vi "OCU_Simple_Main.vi"() -> ()   [LabVIEW 2013]
doc: "To be executed on the Opperator Control Unit (laptop), which communicates to a variety of platforms for the sailbot boat to send missions to complete, override commands, and to monitor the status of the boat and parts of the code run on it. It should be run in parallel with \"Main.vi\" in the cRIO code foler. \n\nCreaded by Victoria Coleman and Elizabeth Mahon (03/14)"
uses:
  cRIO_Code/Data/TypeDefs/UTM Location.ctl
  cRIO_Code/Data/TypeDefs/Constants for OCU Tuning.ctl
  cRIO_Code/Data/TypeDefs/MotorSetup.ctl
  cRIO_Code/Data/TypeDefs/DynamixelSetupInfo.ctl
  cRIO_Code/Data/TypeDefs/Sail Set Suggestions.ctl
  cRIO_Code/Data/TypeDefs/Rudder Set Suggestions.ctl
  cRIO_Code/Logic/Classes/Missions/GenericMission/GenericMission.lvclass
  cRIO_Code/Data/TypeDefs/MainsailPositionIndicator.ctl
  cRIO_Code/Data/TypeDefs/JibPositionIndicator.ctl
  cRIO_Code/Data/TypeDefs/Apparent Wind Point of Sail.ctl
  cRIO_Code/Data/TypeDefs/BoatType.ctl
  cRIO_Code/Logic/Classes/Waypoint/Waypoint.lvclass
  cRIO_Code/Data/TypeDefs/MissionDescription.ctl
  cRIO_Code/Data/TypeDefs/MissionTypeControl.ctl
  cRIO_Code/Data/TypeDefs/Sim_Wind_Speed.ctl
  cRIO_Code/Data/TypeDefs/Sim_Wind_Heading.ctl
  cRIO_Code/Data/TypeDefs/OverrideInformation.ctl
  cRIO_Code/Data/TypeDefs/OverrideMode.ctl
  TypeDef/map_list.ctl
  TypeDef/obstacle_arrays.ctl
  cRIO_Code/Logic/Classes/Obstacle/Obstacle.lvclass
  cRIO_Code/Data/TypeDefs/ObstacleDescription.ctl
  CommandMessages.ctl
  cRIO_Code/Logic/Classes/Missions/GoTo/GoTo.lvclass
  RIO-OCU_Comm/NetworkStreams/Writer/NetworkStreamWriter.lvclass
  RIO-OCU_Comm/NetworkStreams/Reader/NetworkStreamReader.lvclass
panel:
  in  "Main Tab Structure":enum32{"User Interface", "Settings"}(tab)
  in  "Setting Missions with Map Internal Tab":enum32{"Edit Mission", "Monitor Boat"}(tab)
  in  "element":T1 {"North" format="%#_10f"; "East" format="%#_8f"}
  in  "ClearMissionPOI":bool
  in  "CreateMission":bool
  out "Readable Missions":T2[](array[typedef]) {"Points of Interest"."North" format="%#_10f"; "Points of Interest"."East" format="%#_8f"}
  out "Robot Location":T1 {"North" format="%#_10f"; "East" format="%#_8f"}
  out "Rudder Setpoint":T4 min=-0.95 max=0.95 scale=1.0..-1.0
  out "BoatSpeed":dbl(slide) scale=0.0..100.0
  out "Abs Wind Direction":dbl(knob)
  out "Main":T5
  out "Jib":T6
  out "BoatDirection":dbl(knob)
  out "RelWindDirection":T7 scale=0.0..360.0 scale format="%4d"
  out "Set Mission with Map":T8(plugin-control)
  in  "Sim_Wind_Heading":T9
  in  "Sim_Wind_Speed":T10
  out "Reset missions?":bool=TRUE
  out "Missions from Main":refnum<class "GenericMission.lvclass">[](array[class])
  out "Current Missions":refnum<class "GenericMission.lvclass">[](array[class])
  out "Finished Missions":refnum<class "GenericMission.lvclass">[](array[class])
  out "Map display loop counter":i32
  out "User input loop counter":i32
  out "Desired Heading":dbl
  out "Abs Wind Direction":dbl(knob)
  out "Rel Wind Direction":dbl(knob)
  out "Sail Positions":T11 {"MainSailSuggestion" min=0.0 max=1.0; "JibSailSuggestion" min=0.0 max=1.0}
  out "Rudder Setpoint":T4 min=-0.95 max=0.95 scale=1.0..-1.0
  out "BoatDirection":dbl
  out "Final error out":errorcluster
  out "Intermediate\nWaypoints":refnum<class "Waypoint.lvclass">[](array[class])
  in  "Boat Type":T12
  in  "OCU Tuning Constants":T13={"Motor Setting Constant"={"Main Dynamixel Set Data"={"Lower Winch Bound (deg)"=0.0, "Upper Winch Bound (deg)"=1000.0}, "Rudder Dynamixel Set Data"={"Lower Winch Bound (deg)"=30.0, "Upper Winch Bound (deg)"=90.0}, "Jib Dynamixel Set Data"={"Lower Winch Bound (deg)"=0.0, "Upper Winch Bound (deg)"=700.0}}, "Irons Range (deg)"=100.0}
  out "Reader\nConnected?":bool
  out "Writter\nConnected?":bool
  in  "Clear Trace":bool
  in  "Trace Path":bool=TRUE
  out "Sending IDs?":bool
  out "Mission Points of Interest":T1[](array[typedef]) {"North" format="%#_10f"; "East" format="%#_8f"}
  in  "ID# To Delete (miss)":u16
  in  "DeleteMission":bool
  in  "stop":bool
  # "These guys need to be kept even though they aren't human readable, they're used for probing and data passage"
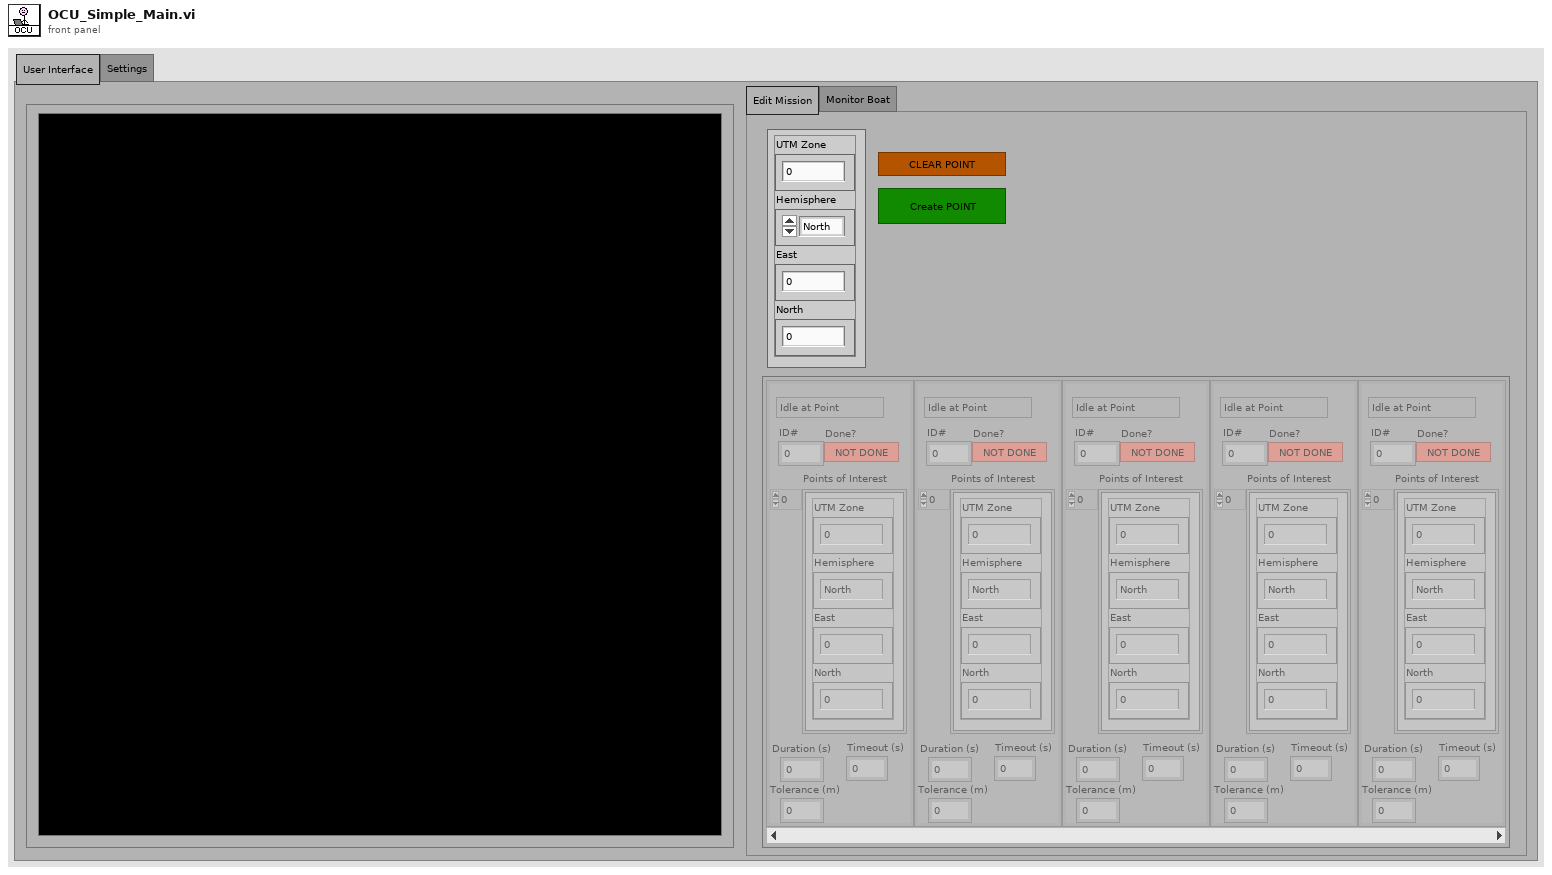
[diagram p1: front panel]
types:
  T1 = typedef "UTM Location.ctl" = cluster{"UTM Zone":dbl, "Hemisphere":enum16{"North", "South"}, "East":dbl, "North":dbl}
  T2 = typedef "MissionDescription.ctl" = cluster{"Duration (s)":dbl, "Timeout (s)":dbl, "Tolerance (m)":dbl, "Mission Type":T3, "Points of Interest":T1[], "ID#":i32, "Done?":bool}
  T3 = typedef "MissionTypeControl.ctl" = enum16{"Idle at Point", "Drive to Waypoint", "Round Buoy to Port", "Round Buoy to Starboard", "Pass Between Buoys", "Station Keeping"}
  T4 = typedef "Rudder Set Suggestions.ctl" = dbl
  T5 = typedef "MainsailPositionIndicator.ctl" = dbl
  T6 = typedef "JibPositionIndicator.ctl" = dbl
  T7 = typedef "Apparent Wind Point of Sail.ctl" = dbl
  T8 = typedef "IMAQ Image.ctl" = refnum<image>
  T9 = typedef "Sim_Wind_Heading.ctl" = dbl
  T10 = typedef "Sim_Wind_Speed.ctl" = dbl
  T11 = typedef "Sail Set Suggestions.ctl" = cluster{"MainSailSuggestion":dbl, "JibSailSuggestion":dbl}
  T12 = typedef "BoatType.ctl" = enum16{"Blackbody Radiation", "ReadLog", "Little boats", "Simulation", "Damn Yankee"}
  T13 = typedef "Constants for OCU Tuning.ctl" = cluster{"Motor Setting Constant":T14, "Irons Range (deg)":dbl}
  T14 = typedef "MotorSetup.ctl" = cluster{"Main Dynamixel Set Data":T15, "Rudder Dynamixel Set Data":T15, "Jib Dynamixel Set Data":T15}
  T15 = typedef "DynamixelSetupInfo.ctl" = cluster{"Lower Winch Bound (deg)":dbl, "Upper Winch Bound (deg)":dbl}
  T16 = typedef "map_list.ctl" = enum16{"Grid", "Olin"}
  T17 = typedef "OverrideInformation.ctl" = cluster{"OverrideMode":T18, "SailSetting":T11, "Rudder Setpoint":T4, "Sim_Wind_Speed":dbl, "Sim_Wind_Heading":dbl}
  T18 = typedef "OverrideMode.ctl" = enum16{"None", "Rudder", "Sails", "Both"}
  T19 = typedef "mission_arrays.ctl" = cluster{"# of Missions":i32, "Readable Missions":T2[], "Mission array":refnum<class "GenericMission.lvclass">[]}
  T20 = typedef "map_metadata.ctl" = cluster{"Meters/pixel":dbl, "Top Left Pixel UTM":T1, "Bottom Right Pixel UTM":T1}
  T21 = typedef "obstacle_arrays.ctl" = cluster{"# of Obstacles":i32, "Obstacle array":refnum<class "Obstacle.lvclass">[], "Readable Obstacles":T22[]}
  T22 = typedef "ObstacleDescription.ctl" = cluster{"ID#":i32, "Obstacle Array":T1[]}
  T23 = typedef "CommandMessages.ctl" = enum16{"Pass", "OverrideMode", "Add mission", "Delete mission", "Add obstacle", "Delete obstacle", "Change constants", "Check mission ID", "Check obstacle ID"}
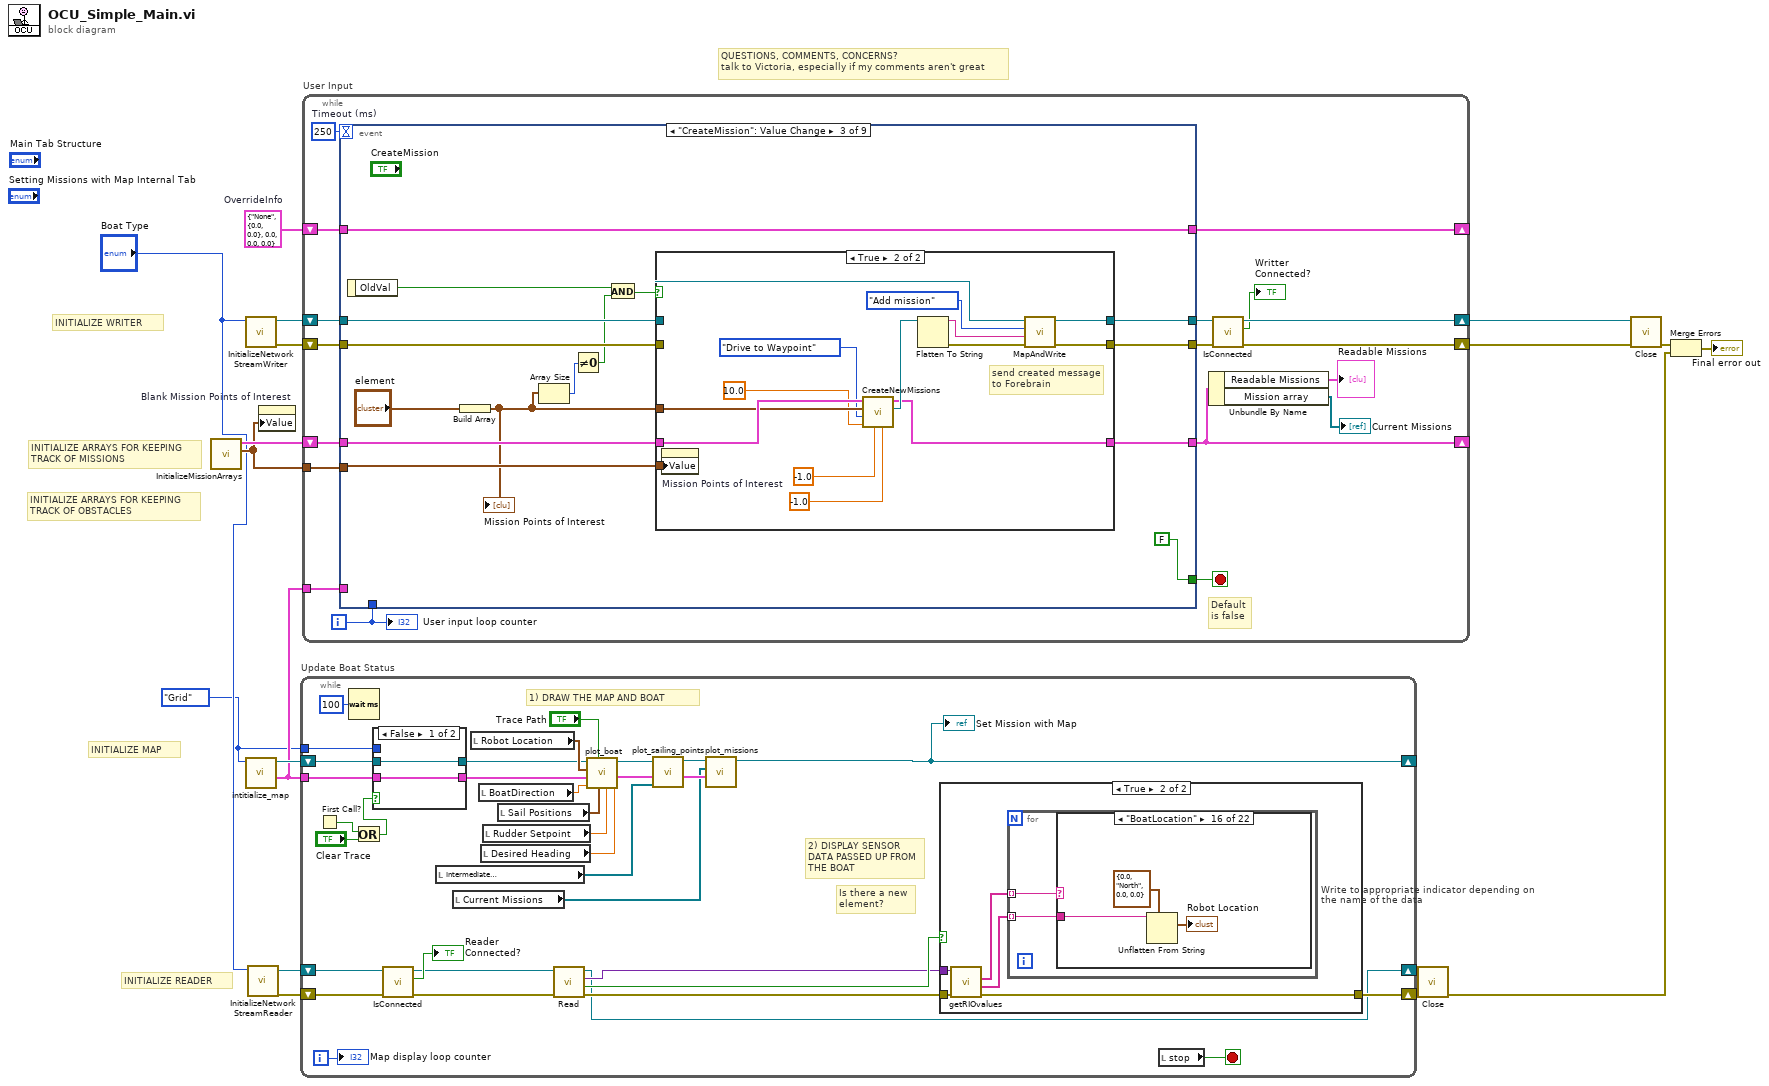
[diagram p0: block diagram]
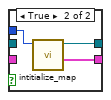
[diagram p2: hidden frame]
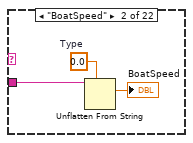
[diagram p5: hidden frame]
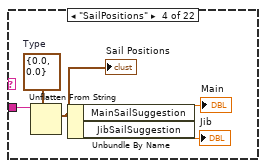
[diagram p7: hidden frame]
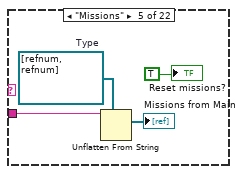
[diagram p8: hidden frame]
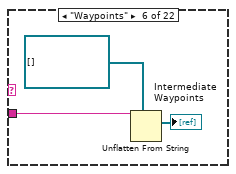
[diagram p9: hidden frame]
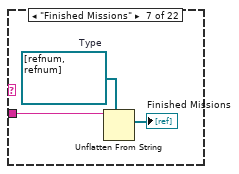
[diagram p10: hidden frame]
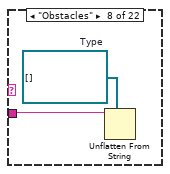
[diagram p11: hidden frame]
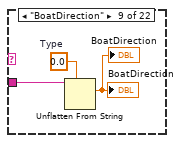
[diagram p12: hidden frame]
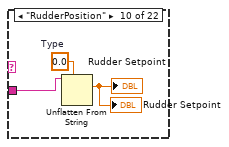
[diagram p13: hidden frame]
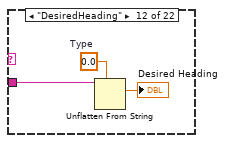
[diagram p15: hidden frame]
diagram:
  w1 = map_list."Grid" ("Map")
  w5 = T17 {"OverrideMode"=enum."None", "SailSetting"={"MainSailSuggestion"=0.0, "JibSailSuggestion"=0.0}, "Rudder Setpoint"=0.0, "Sim_Wind_Speed"=0.0, "Sim_Wind_Heading"=0.0}  # OverrideInfo
  # "INITIALIZE ARRAYS FOR KEEPING TRACK OF OBSTACLES"
  # "INITIALIZE WRITER"
  # "INITIALIZE ARRAYS FOR KEEPING TRACK OF MISSIONS"
  # "INITIALIZE MAP"
  # "INITIALIZE READER"
  # "QUESTIONS, COMMENTS, CONCERNS? \ntalk to Victoria, especially if my comments aren't great"
  n1 = call "InitializeMissionArrays.vi"() -> ("Mission Points of Interest"=w3:T1[], "Initialized Mission Arrays"=w18:T19)  [unwired: 10 in]
  n2 = call "InitializeNetworkStreamWriter.vi"("Boat Type"="Boat Type") -> ("error out"=w15:errorcluster, "NetworkStreamWriter out"=w14:refnum<class "NetworkStreamWriter.lvclass">)  [unwired: 9 in]
  n3 = call "intitialize_map.vi"("Map"=w1) -> ("MapDistanceInfo"=w4:T20, "Map Image Out"=w11:T8)  [unwired: 9 in]
  n4 = call "InitializeNetworkStreamReader.vi"("Boat Type"="Boat Type") -> ("error out"=w9:errorcluster, "NetworkStreamReader out"=w10:refnum<class "NetworkStreamReader.lvclass">)  [unwired: 9 in]
  n5 = property on="Blank Mission Points of Interest" class="Arr (strict)"("Value"=w3) -> ()  [unwired: 2 in, 2 out]
  n6 = while "Update Boat Status" {
    shift-right: [w41] -> w13
    shift-left: w10 -> [w51]
    shift-right: [w47] -> w12
    shift-left: w9 -> [w50]
    tunnel: w4 -> [w36]
    tunnel: w1 -> [w38]
    shift-right: [w23] -> _
    shift-left: w11 -> [w39]
    i -> [w37]
    stop <- w52 stop-if-true
    # "Is there a new element?"
    # "2) DISPLAY SENSOR DATA PASSED UP FROM THE BOAT"
    # "1) DRAW THE MAP AND BOAT"
    n7 = First Call?() -> (First Call?: T/F=w26:bool)
    n8 = Wait (ms)(milliseconds to wait=u32 100) -> ()  [unwired: 1 out]
    n9 = Or(x=w26, y="Clear Trace") -> (x .or. y?=w25:bool)
    n10 = case shown="False" w25 {
      tunnel: w39 -> [w54 _]
      tunnel: [w54 w55] -> w28
      tunnel: w36 -> [w53 _]
      tunnel: [w53 w56] -> w29
      tunnel: w38 -> [_ w57]
      frame False {
      }
      frame True {
        n11 = call "intitialize_map.vi"("Map"=w57) -> ("MapDistanceInfo"=w56:T20, "Map Image Out"=w55:T8)  [unwired: 9 in]
      }
    }
    n12 = call "IsConnected.vi"("error in (no error)"=w50, "NetworkStreamReader in"=w51) -> ("error out"=w45:errorcluster, "Connected?"=→"Reader\nConnected?":bool, "NetworkStreamReader out"=w46:refnum<class "NetworkStreamReader.lvclass">)  [unwired: 7 in]
    n13 = local read "Intermediate\nWaypoints"() -> (w22:refnum<class "Waypoint.lvclass">[])
    n14 = local read "Current Missions"() -> (w19:refnum<class "GenericMission.lvclass">[])
    n15 = local read "Robot Location"() -> (w32:T1)
    n16 = local read "BoatDirection"() -> (w34:dbl)
    n17 = local read "Desired Heading"() -> (w24:dbl)
    n18 = local read "Rudder Setpoint"() -> (w33:T4)
    n19 = local read "Sail Positions"() -> (w35:T11)
    n20 = call "Read.vi"("error in (no error)"=w45, "NetworkStreamReader in"=w46) -> ("error out"=w44:errorcluster, "New element?"=w43:bool, "element"=w42:variant, "NetworkStreamReader out"=w41:refnum<class "NetworkStreamReader.lvclass">)  [unwired: 5 in, 1 out]
    n21 = call "plot_boat.vi"("Desired Heading"=w24, "Rudder Setpoint"=w33, "Sail Setpoints"=w35, "Trace Path"="Trace Path", "Heading"=w34, "MapDistanceInfo"=w29, "UTM Location"=w32, "Map in"=w28) -> ("MapDistanceInfo OUT"=w30:T20, "Map Out"=w31:T8)  [unwired: 1 in, 1 out]
    n22 = call "plot_sailing_points.vi"("Intermediate\nWaypoints"=w22, "MapDistanceInfo"=w30, "Map in"=w31) -> ("MapDistanceInfo OUT"=w21:T20, "Map Out"=w20:T8)  [unwired: 6 in, 1 out]
    n23 = call "plot_missions.vi"("MapDistanceInfo"=w21, "Missions"=w19, "Map in"=w20) -> ("Map Out"=w23:T8)  [unwired: 6 in, 2 out]
    "Set Mission with Map" <- w23
    n24 = case shown="True" w43 {
      tunnel: [w58 w61] -> w47
      tunnel: w44 -> [w58 w60]
      tunnel: w42 -> [_ w59]
      frame False {
      }
      frame True {
        n25 = call "getRIOvalues.vi"("error in"=w60, "element"=w59) -> ("error out"=w61:errorcluster, "data"=w62:string[], "names"=w63:string[])  [unwired: 7 in]
        n26 = for "Write to appropriate indicator depending on the name of the data" {
          tunnel: w63 -> [w65] mode=indexing
          tunnel: w62 -> [w64] mode=indexing
          n27 = case shown="\"BoatLocation\"" w65 {
            tunnel: w64 -> [_ w66 _ w73 w76 w80 w83 w84 w88 w91 _ w92 _ _ _ w97 _ _ _ w99 w103 _]
            frame Default {
              # "unknown name"
            }
            frame "BoatSpeed" {
              w68 = 0.0  # Type
              n28 = Unflatten From String(type=w68, binary string=w66) -> (value=→"BoatSpeed":dbl)  [unwired: 3 in, 2 out]
            }
            frame "WindSpeed" {
            }
            frame "SailPositions" {
              w72 = T11 {"MainSailSuggestion"=0.0, "JibSailSuggestion"=0.0}  # Type
              n29 = Unflatten From String(type=w72, binary string=w73) -> (value=w71:T11)  [unwired: 3 in, 2 out]
              "Sail Positions" <- w71
              n30 = Unbundle By Name(w71) -> ("MainSailSuggestion"=→"Main":dbl, "JibSailSuggestion"=→"Jib":dbl)
            }
            frame "Missions" {
              w77 = refnum<class "GenericMission.lvclass">[] [refnum, refnum]  # Type
              n31 = Unflatten From String(type=w77, binary string=w76) -> (value=→"Missions from Main":refnum<class "GenericMission.lvclass">[])  [unwired: 3 in, 2 out]
              "Reset missions?" <- TRUE
            }
            frame "Waypoints" {
              n32 = Unflatten From String(type=refnum<class "Waypoint.lvclass">[] [] ("elements"), binary string=w80) -> (value=→"Intermediate\nWaypoints":refnum<class "Waypoint.lvclass">[])  [unwired: 3 in, 2 out]
            }
            frame "Finished Missions" {
              w82 = refnum<class "GenericMission.lvclass">[] [refnum, refnum]  # Type
              n33 = Unflatten From String(type=w82, binary string=w83) -> (value=→"Finished Missions":refnum<class "GenericMission.lvclass">[])  [unwired: 3 in, 2 out]
            }
            frame "Obstacles" {
              w85 = refnum<class "Obstacle.lvclass">[] []  # Type
              n34 = Unflatten From String(type=w85, binary string=w84) -> ()  [unwired: 3 in, 3 out]
            }
            frame "BoatDirection" {
              w87 = 0.0  # Type
              n35 = Unflatten From String(type=w87, binary string=w88) -> (value=→"BoatDirection" →"BoatDirection":dbl)  [unwired: 3 in, 2 out]
            }
            frame "RudderPosition" {
              w90 = T4 0.0  # Type
              n36 = Unflatten From String(type=w90, binary string=w91) -> (value=→"Rudder Setpoint" →"Rudder Setpoint":T4)  [unwired: 3 in, 2 out]
            }
            frame "SimWindSpeed(m/s)" {
            }
            frame "DesiredHeading" {
              w94 = 0.0  # Type
              n37 = Unflatten From String(type=w94, binary string=w92) -> (value=→"Desired Heading":dbl)  [unwired: 3 in, 2 out]
            }
            frame "RudderForce" {
            }
            frame "BatteryVoltage" {
            }
            frame "StayForces" {
            }
            frame "BoatLocation" {
              n38 = Unflatten From String(type=T1 {"UTM Zone"=0.0, "Hemisphere"=enum."North", "East"=0.0, "North"=0.0} ("UTM Location"), binary string=w97) -> (value=→"Robot Location":T1)  [unwired: 3 in, 2 out]
            }
            frame "Pitch" {
            }
            frame "Roll" {
            }
            frame "RateOfTurn" {
            }
            frame "RelWindDirection" {
              w100 = 0.0  # Type
              n39 = Unflatten From String(type=w100, binary string=w99) -> (value=→"Rel Wind Direction" →"RelWindDirection":dbl)  [unwired: 3 in, 2 out]
            }
            frame "AbsWindDirection" {
              w102 = 0.0  # Type
              n40 = Unflatten From String(type=w102, binary string=w103) -> (value=→"Abs Wind Direction" →"Abs Wind Direction":dbl)  [unwired: 3 in, 2 out]
            }
            frame "DynamixelTorques" {
            }
          }
        }
      }
    }
    n41 = local read "stop"() -> (w52:bool)
    "Map display loop counter" <- w37
  }
  n42 = while "User Input" {
    shift-right: [w107] -> _
    shift-left: w18 -> [w121]
    shift-right: [w115] -> w16
    shift-left: w15 -> [w119]
    shift-right: [w116] -> w17
    shift-left: w14 -> [w118]
    shift-right: [w113] -> _
    shift-left: w5 -> [w112]
    tunnel: w4 -> [w110]
    tunnel: w3 -> [w109]
    i -> [w105]
    stop <- w120 stop-if-true
    w108 = 250  # Timeout (ms)
    # "Default is false"
    n43 = event shown="[2] \"CreateMission\": Value Change" {
      selector: _ -> [_ _ _ _ _ _ _ _ _]
      dyn-events: _ -> [_ _ _ _ _ _ _ _ _]
      timeout: w108 -> [_ _ _ _ _ _ _ _ _]
      tunnel: w121 -> [w137 w152 w170 w189 w204 w210 w218 w223 w232]
      tunnel: [FALSE TRUE FALSE FALSE _ _ _ _ _] -> w120
      tunnel: [w127 w151 w163 w197 w201 w206 w220 w222 w234] -> w111
      tunnel: w118 -> [w131 w154 w168 w195 w200 w209 w221 w227 w237]
      tunnel: w119 -> [w132 w151 w167 w196 w203 w213 w220 w228 _]
      tunnel: [w128 w154 w166 w194 w200 w209 w221 w226 w235] -> w117
      tunnel: [w140 w153 w165 w193 w199 w211 w219 w224 w233] -> w113
      tunnel: w112 -> [w140 w153 w165 w193 w199 w211 w219 w224 w240]
      tunnel: w110 -> [_ _ _ _ _ w214 _ _ _]
      tunnel: w109 -> [_ _ w164 _ w205 _ _ _ _]
      tunnel: [w124 w152 w158 w192 w204 w210 w218 w223 w232] -> w107
      tunnel: w105 -> [w130 _ _ _ _ _ _ _ _]
      event Timeout {
        n44 = event-data() -> ()  [unwired: 1 in, 1 out]
        n45 = First Call?() -> (First Call?: T/F=w138:bool)
        n46 = Unbundle By Name(w137) -> ("# of Missions"=w129:i32, "Mission array"=w136:refnum<class "GenericMission.lvclass">[], "Readable Missions"=w135:T2[])
        n47 = case shown="True" w138 {
          tunnel: [w147 w148] -> w139
          frame False {
            n48 = local read "Finished Missions"() -> (w147:refnum<class "GenericMission.lvclass">[])
          }
          frame True {
            w150 = refnum<class "GenericMission.lvclass"> refnum  # Initializer array for Finished Missions
            n49 = Initialize Array(w150, 0 ("dimension size")) -> (w148:refnum<class "GenericMission.lvclass">[])
            n50 = local write "Finished Missions"(w148) -> ()
          }
        }
        n51 = call "SendMissionObstacleIDs.vi"("Loop counter"=w130, "error in (no error)"=w132, "# of Missions"=w129, "Obstacle Arrays Cluster"=T21 {"# of Obstacles"=0, "Obstacle array"=[], "Readable Obstacles"=[]}, "NetworkStreamWriter in"=w131) -> ("error out"=w127:errorcluster, "Sending IDs?"=→"Sending IDs?":bool, "NetworkStreamWriter out"=w128:refnum<class "NetworkStreamWriter.lvclass">)  [unwired: 4 in]
        n52 = call "mark_finished_missions.vi"("Finished Missions"=w139, "Current Missions (human readable)"=w135, "Current Missions"=w136) -> (2:"Current Missions OUT"=w134:T2[], 3:"Current Missions OUT"=w133:refnum<class "GenericMission.lvclass">[])  [unwired: 7 in]
        n53 = Bundle By Name(cluster=w137, "# of Missions"=w129, "Mission array"=w133, "Readable Missions"=w134) -> (w125:T19)
        n54 = local read "Reset missions?"() -> (w126:bool)
        n55 = case shown="True" w126 {
          tunnel: w125 -> [w142 w145]
          tunnel: [w142 w144] -> w124
          frame False {
          }
          frame True {
            n56 = local read "Missions from Main"() -> (w143:refnum<class "GenericMission.lvclass">[])
            n57 = local write "Reset missions?"(FALSE ("Reset missions?")) -> ()
            n58 = call "ResetMissionArrays.vi"("Mission Array Replacement"=w143, "Mission Arrays"=w145) -> ("Mission Arrays"=w144:T19)  [unwired: 9 in]
          }
        }
      }
      event "stop": Value Change {
        # "Putting the button in here keeps the code from breaking, leave it here :)\nHas to do with how event structures work"
        n59 = event-data() -> ()  [unwired: 1 in, 2 out]
      }
      event "CreateMission": Value Change {
        n60 = event-data() -> ("OldVal"=w159:bool)  [unwired: 1 in]
        n61 = Build Array("element") -> (w157:T1[])
        "Mission Points of Interest" <- w157
        n62 = Array Size(array=w157) -> (size(s)=w162:i32)
        n63 = Not Equal To 0?(x=w162) -> (x != 0?=w160:bool)
        n64 = And(x=w159, y=w160) -> (x .and. y?=w161:bool)
        n65 = case shown="True" w161 {
          tunnel: w170 -> [w171 w181]
          tunnel: [w171 w177] -> w158
          tunnel: [w173 w183] -> w163
          tunnel: w168 -> [w172 w186]
          tunnel: w167 -> [w173 _]
          tunnel: [w172 w184] -> w166
          tunnel: w164 -> [_ w176]
          tunnel: w157 -> [_ w180]
          frame False {
          }
          frame True {
            # "send created message to Forebrain"
            n66 = property on="Mission Points of Interest" class="Arr (strict)"("Value"=w176) -> ()  [unwired: 2 in, 2 out]
            n67 = call "CreateNewMissions.vi"("Timeout (s)"=-1.0, "Duration (s)\n[For in-box mission]"=-1.0 ("Duration (s)\n[For in-box mission]"), "Tolerance (m)"=10.0, "Mission Type"=MissionTypeControl."Drive to Waypoint", "Points of Interest"=w180, "Initialized Mission Arrays"=w181) -> ("New Mission OUT"=w178:refnum<class "GenericMission.lvclass">, "Mission Array Cluster"=w177:T19)  [unwired: 4 in]
            n68 = Flatten To String(anything=w178) -> (data string=w185:string, error out=w182:errorcluster)  [unwired: 3 in, 1 out]
            n69 = call "MapAndWrite.vi"("error in (no error)"=w182, "String_Cast_of_Info"=w185, "Commands"=CommandMessages."Add mission", "NetworkStreamWriter in"=w186) -> ("error out"=w183:errorcluster, "NetworkStreamWriter out"=w184:refnum<class "NetworkStreamWriter.lvclass">)  [unwired: 2 in]
          }
        }
      }
      event "DeleteMission": Value Change {
        n70 = event-data() -> ("OldVal"=w191:bool)  [unwired: 1 in]
        n71 = call "DeleteMission.vi"("OldVal"=w191, "ID# To Delete (miss)"="ID# To Delete (miss)", "error in (no error)"=w196, "Initialized Mission Arrays in"=w189, "NetworkStreamWriter in"=w195) -> ("error out"=w197:errorcluster, "Initialized Mission Arrays out"=w192:T19, "NetworkStreamWriter out"=w194:refnum<class "NetworkStreamWriter.lvclass">)  [unwired: 4 in]
      }
      event "ClearMissionPOI": Value Change {
        n72 = event-data() -> ()  [unwired: 1 in, 2 out]
        n73 = property on="Setting Missions with Map Internal Tab" class="TabCtl (strict)" props=["Value"](error in=w203) -> (error out=w202:errorcluster)  [unwired: 1 in, 2 out]
        n74 = property on="Mission Points of Interest" class="Arr (strict)"(error in=w202, "Value"=w205) -> (error out=w201:errorcluster)  [unwired: 1 in, 1 out]
      }
      event "Set Mission with Map": Mouse Up {
        n75 = event-data() -> ()  [unwired: 1 in, 3 out]
        n76 = property on="Set Mission with Map" class="ImageControl"(error in=w213) -> (error out=w206:errorcluster, "Last Mouse Position"=w212:cluster{"X":i32, "Y":i32})  [unwired: 1 in, 1 out]
        n77 = property on="Setting Missions with Map Internal Tab" class="TabCtl (strict)"() -> ("Value"=w208:enum32{"Edit Mission", "Monitor Boat"})  [unwired: 2 in, 2 out]
        n78 = call "ImageUTMPosition.vi"("Pixel Coordinates"=w212, "MapDistanceInfo"=w214) -> ("output cluster"=w207:T1)  [unwired: 9 in]
        n79 = case shown="\"Edit Mission\"" w208 {
          tunnel: w207 -> [_ w215]
          frame Default {
          }
          frame "Edit Mission" {
            n80 = property on="Mission Points of Interest" class="Arr (strict)"() -> ("Value"=w216:T1[])  [unwired: 2 in, 2 out]
            n81 = Build Array (concatenate)(w216, w215) -> (w217:T1[])
            n82 = property on="Mission Points of Interest" class="Arr (strict)"("Value"=w217) -> ()  [unwired: 2 in, 2 out]
          }
        }
      }
      event Key Down; Key Repeat {
        n83 = event-data() -> ()  [unwired: 1 in, 1 out]
      }
      event Value Change {
        n84 = event-data() -> ()  [unwired: 1 in, 2 out]
        n85 = Flatten To String(anything="OCU Tuning Constants", error in (no error)=w228) -> (data string=w230:string, error out=w229:errorcluster)  [unwired: 2 in, 1 out]
        n86 = call "MapAndWrite.vi"("error in (no error)"=w229, "String_Cast_of_Info"=w230, "Commands"=CommandMessages."Change constants", "NetworkStreamWriter in"=w227) -> ("error out"=w222:errorcluster, "NetworkStreamWriter out"=w226:refnum<class "NetworkStreamWriter.lvclass">)  [unwired: 2 in]
      }
      event Value Change {
        n87 = event-data() -> ()  [unwired: 1 in, 6 out]
        n88 = Bundle By Name(cluster=w240, "Sim_Wind_Speed"="Sim_Wind_Speed", "Sim_Wind_Heading"="Sim_Wind_Heading") -> (w233:T17)
        n89 = Flatten To String(anything=w233) -> (data string=w239:string, error out=w236:errorcluster)  [unwired: 3 in, 1 out]
        n90 = call "MapAndWrite.vi"("error in (no error)"=w236, "String_Cast_of_Info"=w239, "Commands"=CommandMessages."OverrideMode", "NetworkStreamWriter in"=w237) -> ("error out"=w234:errorcluster, "NetworkStreamWriter out"=w235:refnum<class "NetworkStreamWriter.lvclass">)  [unwired: 2 in]
      }
    }
    n91 = Unbundle By Name(w107) -> ("Readable Missions"=→"Readable Missions":T2[], "Mission array"=→"Current Missions":refnum<class "GenericMission.lvclass">[])
    n92 = call "IsConnected.vi"("error in (no error)"=w111, "NetworkStreamWriter in"=w117) -> ("error out"=w115:errorcluster, "Connected?"=→"Writter\nConnected?":bool, "NetworkStreamWriter out"=w116:refnum<class "NetworkStreamWriter.lvclass">)  [unwired: 7 in]
    "User input loop counter" <- w105
  }
  n93 = call "Close.vi"("error in (no error)"=w12, "NetworkStreamReader in"=w13) -> ("error out"=w7:errorcluster)  [unwired: 9 in]
  n94 = call "Close.vi"("error in (no error)"=w16, "NetworkStreamWriter in"=w17) -> ("error out"=w8:errorcluster)  [unwired: 9 in]
  n95 = Merge Errors(w8, w7) -> (→"Final error out":errorcluster)
